vi "Reinitialize All.vi"(8 "error in (no error)":errorcluster, 10 "Initialize":bool, 11 "Create Project View in":refnum<class "Create Project View.lvclass">) -> (0 "error out":errorcluster, 3 "Create Project View out":refnum<class "Create Project View.lvclass">)   [LabVIEW 2013, in "Create Project View.lvlib" / "Create Project View.lvclass"]
uses:
  Create Project View.lvclass
  Create Project View.lvclass/Create Project View.ctl
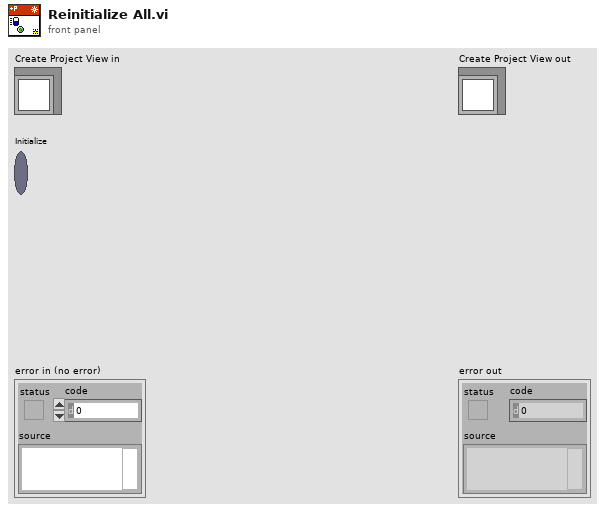
[diagram p1: front panel]
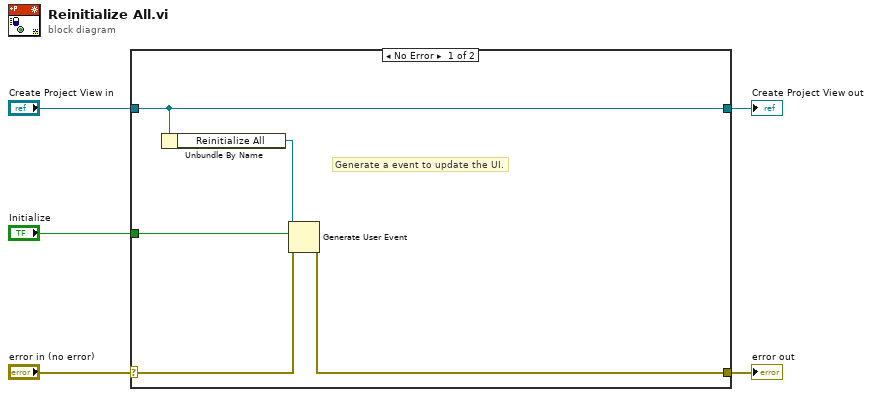
[diagram p0: block diagram]
diagram:
  n1 = case shown="No Error" "error in (no error)" {
    selector: "error in (no error)" -> [w7 w12]
    tunnel: [w6 w12] -> w4
    tunnel: [w10 w11] -> w2
    tunnel: "Create Project View in" -> [w10 w11]
    tunnel: "Initialize" -> [w8 _]
    frame No Error {
      # "Generate a event to update the UI."
      n2 = Unbundle By Name(w10) -> ("Reinitialize All"=w9:refnum<user-event>)
      n3 = Generate User Event(user event=w9, event data cluster=w8, error in=w7) -> (error out=w6:errorcluster)  [unwired: 1 in, 1 out]
    }
    frame Error {
    }
  }
  "error out" <- w4
  "Create Project View out" <- w2
